vi "Arm Logic.vi"(0 "Manual Up":bool, 1 "Manual Down":bool, 2 "Load":bool, 3 "Switch":bool, 4 "Exchange":bool, 5 "Scale Low":bool, 6 "Scale Mid":bool, 7 "Scale High":bool, 9 "Stow":bool, 10 "Reset State Machine":bool, 11 "Climb":bool, 13 "Visited Disabled":bool) -> (17 "Climb Out":bool, 18 "Portal Out":bool, 19 "Stow Out":bool, 20 "Manual Up Out":bool, 21 "Manual Down Out":bool, 22 "Load Out":bool, 23 "Switch Out":bool, 24 "Exchange Out":bool, 25 "Scale Low Out":bool, 26 "Scale Mid Out":bool, 27 "Scale High Out":bool)   [LabVIEW 2017]
uses:
  Lift Portal Switch Setpoints.ctl
panel:
  in  "Portal":bool
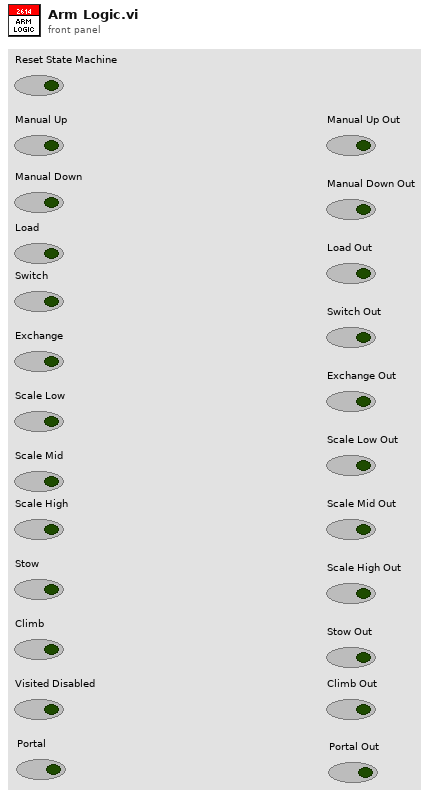
[diagram p1: front panel]
types:
  T1 = typedef "Lift Portal Switch Setpoints.ctl" = enum16{"Waiting for First", "Load", "Portal"}
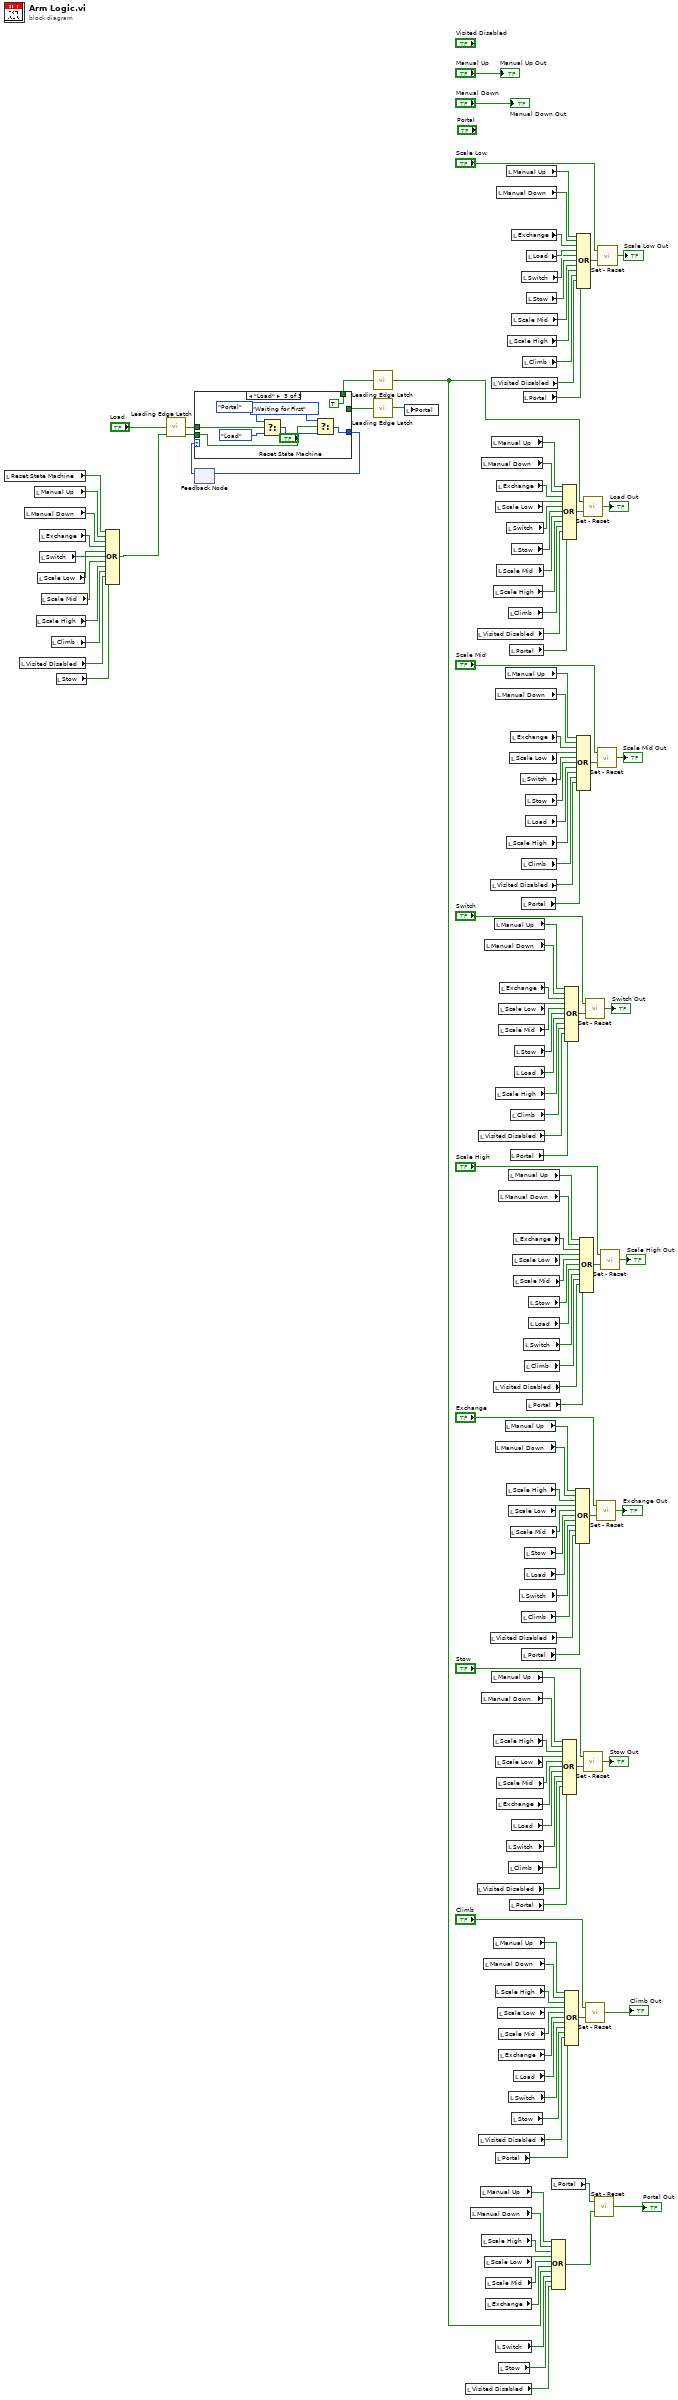
[diagram p0: block diagram]
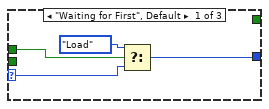
[diagram p2: hidden frame]
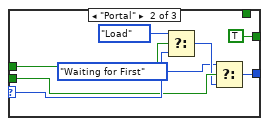
[diagram p3: hidden frame]
diagram:
  n1 = local read "Reset State Machine"() -> (w1:bool)
  n2 = local read "Visited Disabled"() -> (w4:bool)
  n3 = local read "Manual Down"() -> (w6:bool)
  n4 = local read "Manual Up"() -> (w5:bool)
  n5 = local read "Scale High"() -> (w11:bool)
  n6 = local read "Scale Low"() -> (w9:bool)
  n7 = local read "Exchange"() -> (w7:bool)
  n8 = local read "Switch"() -> (w8:bool)
  n9 = local read "Scale Mid"() -> (w10:bool)
  n10 = local read "Climb"() -> (w12:bool)
  n11 = local read "Stow"() -> (w3:bool)
  n12 = Compound Arithmetic op=OR(w1, w5, w6, w7, w8, w9, w10, w11, w12, w4, w3) -> (w2:bool)
  n13 = call "Leading Edge Latch.vi"("Input"="Load") -> ("Output"=w40:bool)
  n14 = feedback #1() -> (w37:T1)  [unwired: 1 in]
  n15 = case shown="\"Load\"" w37 {
    selector: w37 -> [w147 w156 _]
    tunnel: w40 -> [w148 w157 w162]
    tunnel: w2 -> [_ w155 w159]
    tunnel: [_ TRUE _] -> w36
    tunnel: [_ _ TRUE] -> w39
    tunnel: [w146 w151 w158] -> w38
    frame "Waiting for First", Default {
      n16 = Select(t=Lift_Portal_Switch_Setpoints."Load" ("Portal-Switch"), s=w148, f=w147) -> (s? t:f=w146:T1)
    }
    frame "Portal" {
      n17 = Select(t=Lift_Portal_Switch_Setpoints."Load", s=w157, f=w156) -> (s? t:f=w154:T1)
      n18 = Select(t=Lift_Portal_Switch_Setpoints."Waiting for First", s=w155, f=w154) -> (s? t:f=w151:T1)
    }
    frame "Load" {
      n19 = Select(t=Lift_Portal_Switch_Setpoints."Portal" ("Portal-Switch"), s=w162, f=Lift_Portal_Switch_Setpoints."Load") -> (s? t:f=w160:T1)
      n20 = Select(t=Lift_Portal_Switch_Setpoints."Waiting for First", s=w159, f=w160) -> (s? t:f=w158:T1)
    }
  }
  n21 = feedback-in #1(w38) -> ()
  n22 = call "Leading Edge Latch.vi"("Input"=w39) -> ("Output"=w13:bool)
  n23 = call "Leading Edge Latch.vi"("Input"=w36) -> ("Output"=w34:bool)
  n24 = local write "Portal"(w34) -> ()
  n25 = local read "Visited Disabled"() -> (w25:bool)
  n26 = local read "Manual Down"() -> (w27:bool)
  n27 = local read "Visited Disabled"() -> (w121:bool)
  n28 = local read "Visited Disabled"() -> (w129:bool)
  n29 = local read "Visited Disabled"() -> (w123:bool)
  n30 = local read "Visited Disabled"() -> (w132:bool)
  n31 = local read "Manual Up"() -> (w26:bool)
  n32 = local read "Manual Down"() -> (w114:bool)
  n33 = local read "Manual Down"() -> (w106:bool)
  n34 = local read "Scale High"() -> (w33:bool)
  n35 = local read "Manual Down"() -> (w104:bool)
  n36 = local read "Manual Down"() -> (w112:bool)
  n37 = local read "Scale Low"() -> (w32:bool)
  n38 = local read "Scale Mid"() -> (w31:bool)
  n39 = local read "Exchange"() -> (w30:bool)
  n40 = local read "Visited Disabled"() -> (w127:bool)
  n41 = local read "Visited Disabled"() -> (w122:bool)
  n42 = local read "Visited Disabled"() -> (w120:bool)
  n43 = local read "Manual Up"() -> (w115:bool)
  n44 = local read "Manual Up"() -> (w107:bool)
  n45 = local read "Scale High"() -> (w88:bool)
  n46 = local read "Scale High"() -> (w55:bool)
  n47 = local read "Visited Disabled"() -> (w125:bool)
  n48 = local read "Manual Up"() -> (w105:bool)
  n49 = local read "Manual Up"() -> (w113:bool)
  n50 = local read "Manual Down"() -> (w108:bool)
  n51 = local read "Scale High"() -> (w42:bool)
  n52 = local read "Scale Low"() -> (w92:bool)
  n53 = local read "Manual Down"() -> (w116:bool)
  n54 = local read "Scale High"() -> (w72:bool)
  n55 = local read "Scale Low"() -> (w54:bool)
  n56 = local read "Portal"() -> (w22:bool)
  n57 = local read "Switch"() -> (w29:bool)
  n58 = local read "Manual Down"() -> (w118:bool)
  n59 = local read "Exchange"() -> (w93:bool)
  n60 = local read "Scale Mid"() -> (w89:bool)
  n61 = local read "Scale Mid"() -> (w53:bool)
  n62 = local read "Exchange"() -> (w52:bool)
  n63 = local read "Scale Low"() -> (w43:bool)
  n64 = local read "Scale Low"() -> (w76:bool)
  n65 = local read "Scale Mid"() -> (w75:bool)
  n66 = local read "Manual Down"() -> (w110:bool)
  n67 = local read "Scale Mid"() -> (w44:bool)
  n68 = local read "Exchange"() -> (w45:bool)
  n69 = local read "Stow"() -> (w28:bool)
  n70 = local read "Exchange"() -> (w77:bool)
  n71 = local read "Manual Up"() -> (w109:bool)
  n72 = local read "Manual Up"() -> (w117:bool)
  n73 = local read "Manual Up"() -> (w119:bool)
  n74 = local read "Scale High"() -> (w62:bool)
  n75 = local read "Switch"() -> (w91:bool)
  n76 = local read "Scale High"() -> (w80:bool)
  n77 = local read "Switch"() -> (w50:bool)
  n78 = local read "Scale High"() -> (w95:bool)
  n79 = local read "Climb"() -> (w87:bool)
  n80 = local read "Climb"() -> (w49:bool)
  n81 = local read "Manual Up"() -> (w111:bool)
  n82 = local read "Scale Low"() -> (w61:bool)
  n83 = local read "Switch"() -> (w47:bool)
  n84 = local read "Portal"() -> (w16:bool)
  n85 = local read "Scale Low"() -> (w84:bool)
  n86 = local read "Portal"() -> (w21:bool)
  n87 = local read "Portal"() -> (w18:bool)
  n88 = local read "Scale Mid"() -> (w60:bool)
  n89 = local read "Exchange"() -> (w85:bool)
  n90 = local read "Climb"() -> (w71:bool)
  n91 = local read "Exchange"() -> (w100:bool)
  n92 = local read "Scale Mid"() -> (w96:bool)
  n93 = local read "Stow"() -> (w90:bool)
  n94 = local read "Load"() -> (w51:bool)
  n95 = local read "Stow"() -> (w48:bool)
  n96 = local read "Scale Low"() -> (w68:bool)
  n97 = local read "Exchange"() -> (w69:bool)
  n98 = local read "Scale Mid"() -> (w67:bool)
  n99 = local read "Load"() -> (w46:bool)
  n100 = local read "Stow"() -> (w74:bool)
  n101 = local read "Load"() -> (w73:bool)
  n102 = local read "Switch"() -> (w57:bool)
  n103 = local read "Switch"() -> (w83:bool)
  n104 = local read "Switch"() -> (w98:bool)
  n105 = local read "Climb"() -> (w56:bool)
  n106 = local read "Climb"() -> (w79:bool)
  n107 = local read "Portal"() -> (w17:bool)
  n108 = local read "Portal"() -> (w20:bool)
  n109 = local read "Climb"() -> (w94:bool)
  n110 = local read "Portal"() -> (w15:bool)
  n111 = local read "Switch"() -> (w64:bool)
  n112 = local read "Climb"() -> (w63:bool)
  n113 = local read "Stow"() -> (w59:bool)
  n114 = local read "Load"() -> (w58:bool)
  n115 = local read "Stow"() -> (w82:bool)
  n116 = local read "Load"() -> (w81:bool)
  n117 = local read "Load"() -> (w99:bool)
  n118 = local read "Stow"() -> (w97:bool)
  n119 = local read "Portal"() -> (w19:bool)
  n120 = local read "Stow"() -> (w66:bool)
  n121 = local read "Load"() -> (w65:bool)
  n122 = Compound Arithmetic op=OR(w26, w27, w33, w32, w31, w30, w13, w29, w28, w25) -> (w23:bool)
  n123 = local read "Portal"() -> (w14:bool)
  n124 = Compound Arithmetic op=OR(w115, w114, w93, w92, w91, w90, w89, w88, w87, w121, w16) -> (w103:bool)
  n125 = Compound Arithmetic op=OR(w107, w106, w55, w54, w53, w52, w51, w50, w49, w129, w21) -> (w131:bool)
  n126 = Compound Arithmetic op=OR(w113, w112, w77, w76, w75, w74, w73, w72, w71, w123, w18) -> (w101:bool)
  n127 = Compound Arithmetic op=OR(w105, w104, w42, w43, w44, w45, w46, w47, w48, w132, w22) -> (w138:bool)
  n128 = Compound Arithmetic op=OR(w109, w108, w62, w61, w60, w59, w58, w57, w56, w127, w20) -> (w126:bool)
  n129 = Compound Arithmetic op=OR(w117, w116, w85, w84, w83, w82, w81, w80, w79, w122, w17) -> (w102:bool)
  n130 = Compound Arithmetic op=OR(w119, w118, w100, w99, w98, w97, w96, w95, w94, w120, w15) -> (w136:bool)
  n131 = Compound Arithmetic op=OR(w111, w110, w69, w68, w67, w66, w65, w64, w63, w125, w19) -> (w124:bool)
  n132 = call "Set - Reset.vi"("Reset"=w103, "Set"=w13) -> ("Output"=→"Load Out":bool)
  n133 = call "Set - Reset.vi"("Reset"=w131, "Set"="Stow") -> ("Output"=→"Stow Out":bool)
  n134 = call "Set - Reset.vi"("Reset"=w101, "Set"="Switch") -> ("Output"=→"Switch Out":bool)
  n135 = call "Set - Reset.vi"("Reset"=w138, "Set"="Climb") -> ("Output"=→"Climb Out":bool)
  n136 = call "Set - Reset.vi"("Reset"=w23, "Set"=w14) -> ("Output"=→"Portal Out":bool)
  n137 = call "Set - Reset.vi"("Reset"=w126, "Set"="Exchange") -> ("Output"=→"Exchange Out":bool)
  n138 = call "Set - Reset.vi"("Reset"=w102, "Set"="Scale Mid") -> ("Output"=→"Scale Mid Out":bool)
  n139 = call "Set - Reset.vi"("Reset"=w136, "Set"="Scale Low") -> ("Output"=→"Scale Low Out":bool)
  n140 = call "Set - Reset.vi"("Reset"=w124, "Set"="Scale High") -> ("Output"=→"Scale High Out":bool)
  "Manual Up Out" <- "Manual Up"
  "Manual Down Out" <- "Manual Down"
